vi "PMS7003_init_subVi.vi"(8 "error in":errorcluster, 10 "Init":bool, 11 "VISA Refnum in":refnum<visa-resource-name>) -> (0 "error out":errorcluster, 3 "VISA Refnum out":refnum<visa-resource-name>)   [LabVIEW 2019]
uses:
  <vilib>/Instr/_visa.llb/VISA Configure Serial Port (Instr).vi
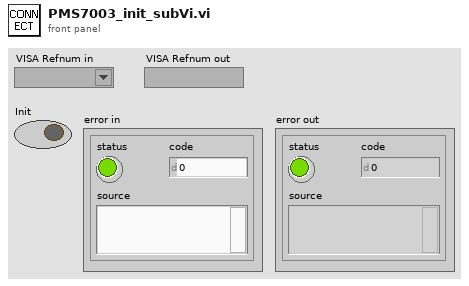
[diagram p1: front panel]
types:
  T1 = cluster{"baud rate":u32, "data bits":u16, "parity":enum16{"None", "Odd", "Even", "Mark", "Space"}, "stop bits":u16, "flow control":u16}
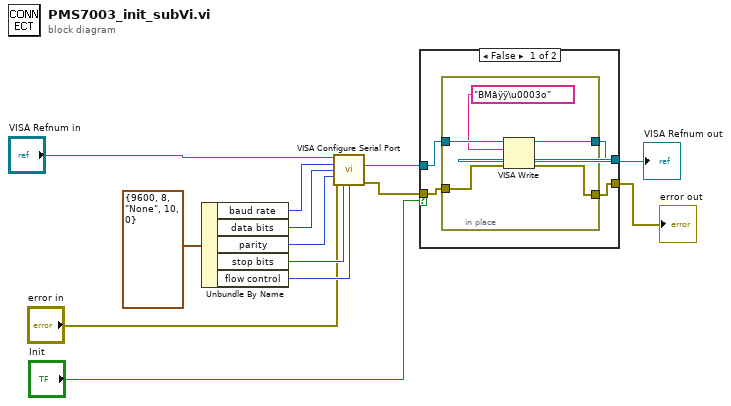
[diagram p0: block diagram]
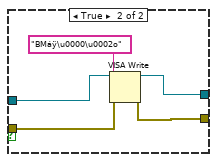
[diagram p2: hidden frame]
diagram:
  n1 = Unbundle By Name(T1 {"baud rate"=9600, "data bits"=8, "parity"=enum."None", "stop bits"=10, "flow control"=0} ("input cluster")) -> ("baud rate"=w6:u32, "data bits"=w5:u16, "parity"=w4:enum16{"None", "Odd", "Even", "Mark", "Space"}, "stop bits"=w3:u16, "flow control"=w7:u16)
  n2 = call-poly "VISA Configure Serial Port"("VISA resource name"="VISA Refnum in", "baud rate (9600)"=w6, "data bits (8)"=w5, "parity (0:none)"=w4, "error in (no error)"="error in", "stop bits (10: 1 bit)"=w3, "flow control (0:none)"=w7) -> ("VISA resource name out"=w8:refnum<visa-resource-name>, "error out"=w9:errorcluster)  [unwired: 3 in, 4 out]
  n3 = case shown="False" "Init" {
    tunnel: w8 -> [w17 w25]
    tunnel: [w14 w27] -> w10
    tunnel: [w15 w26] -> w11
    tunnel: w9 -> [w16 w24]
    frame False {
      n4 = in-place {
        in-place-border: w17 -> [w22]
        in-place-border: w16 -> [w21]
        in-place-border: [w20] -> w15
        in-place-border: [w19] -> w14
        n5 = VISA Write(VISA resource name=w22, write buffer="BMâÿÿ\u0003o", error in (no error)=w21) -> (VISA resource name out=w19:refnum<visa-resource-name>, error out=w20:errorcluster)  [unwired: 1 out]
      }
    }
    frame True {
      n6 = VISA Write(VISA resource name=w25, write buffer="BMáÿ\u0000\u0002o", error in (no error)=w24) -> (VISA resource name out=w27:refnum<visa-resource-name>, error out=w26:errorcluster)  [unwired: 1 out]
    }
  }
  "error out" <- w11
  "VISA Refnum out" <- w10
